vi "Handle Value Change.vi"(5 "VolatusAPI":refnum<class "VolatusAPI.lvclass">, 7 "CtlRef":refnum<vi>, 8 "error in (no error)":errorcluster, 9 "NewVal":variant, 10 "OldVal":variant, 11 "DigitalButtonControl in":refnum<class "DigitalButtonControl.lvclass">) -> (0 "error out":errorcluster, 3 "DigitalButtonControl out":refnum<class "DigitalButtonControl.lvclass">)   [LabVIEW 2023, in "VolatusGUIElements.lvlib" / "DigitalButtonControl.lvclass"]
uses:
  DigitalButtonControl.lvclass
  Volatus/VolatusAPI/VolatusAPI.lvclass
  messages/CmdDigital/Data.ctl
  DigitalButtonControl.lvclass/DigitalButtonControl.ctl
  messages/CmdDigital/Class/Msg.lvclass/Msg.ctl
  Volatus/VolatusAPI/VolatusAPI.lvclass/VolatusAPI.ctl
  messages/CmdDigital/Class/Msg.lvclass
  lv-vecto/Vecto/TCPMessageService/Send Message.vi
  <vilib>/Utility/error.llb/Error Cluster From Error Code.vi
  lv-protoc/LV-Proto/Message/Message.lvclass
  messages/CmdDigital/CmdDigital.lvlib
  VolatusGUI/GUI Element/GUI Element.lvclass
  messages/CmdDigitalMultiple/Class/Msg.lvclass
  C:/dev/volatus/mts-volatus-super/libs/lv-volatus/messages/CmdDigitalMultiple/Class/Msg.lvclass
  C:/dev/volatus/mts-volatus-super/libs/lv-protoc/LV-Proto/Message/Message.lvclass
  C:/dev/volatus/mts-volatus-super/libs/lv-volatus/VolatusGUI/GUI Element/GUI Element.lvclass
  C:/dev/volatus/mts-volatus-super/libs/lv-volatus/VolatusGUIElements/DigitalButtonControl/DigitalButtonControl.lvclass
  C:/dev/volatus/mts-volatus-super/libs/lv-volatus/VolatusGUI/OnValueChangeHandler/OnValueChangeHandler.lvclass
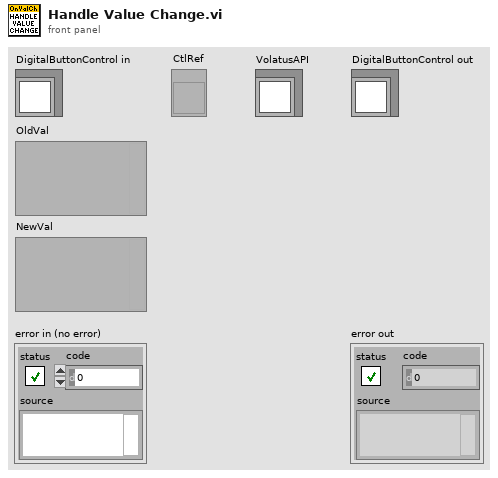
[diagram p1: front panel]
types:
  T1 = typedef "CmdDigital.lvlib/Data.ctl" = cluster{"channel":string, "value":bool}
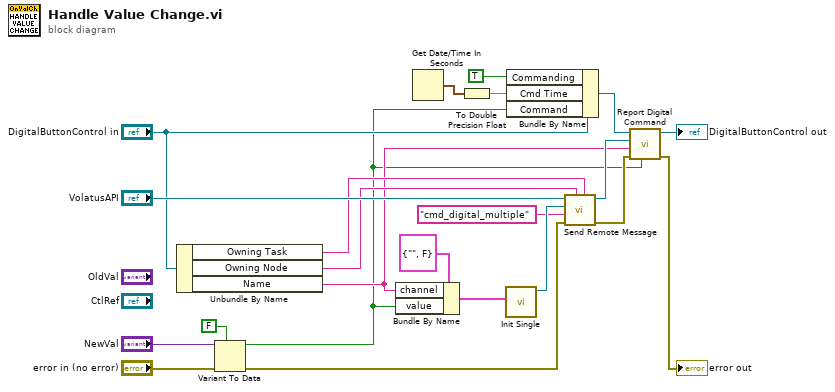
[diagram p0: block diagram]
diagram:
  n1 = Unbundle By Name("DigitalButtonControl in") -> ("Owning Task"=w8:string, "Owning Node"=w7:string, "Name"=w2:string)
  n2 = Variant To Data(error in="error in (no error)", type=FALSE, Variant="NewVal") -> (data=w1:bool, error out=w9:errorcluster)
  n3 = Bundle By Name(cluster=T1 {"channel"="", "value"=FALSE} ("Data"), "channel"=w2, "value"=w1) -> (w18:T1)
  n4 = Get Date/Time In Seconds() -> (seconds since 1Jan1904=w13:timestamp)
  n5 = To Double Precision Float(number=w13) -> (double precision float=w12:dbl)
  n6 = call "Init Single.vi"("value"=w18) -> ("Msg out"=w16:refnum<class "Msg.lvclass">)  [unwired: 10 in]
  n7 = Bundle By Name(cluster="DigitalButtonControl in", "Commanding"=TRUE, "Cmd Time"=w12, "Command"=w1) -> (w14:refnum<class "DigitalButtonControl.lvclass">)
  n8 = call "Send Remote Message.vi"("Target Task (None)"=w8, "Target Name"=w7, "error in (no error)"=w9, "Message Type"="cmd_digital_multiple", "Message"=w16, "VolatusAPI in"="VolatusAPI") -> ("error out"=w5:errorcluster, "VolatusAPI out"=w3:refnum<class "VolatusAPI.lvclass">)  [unwired: 4 in]
  n9 = call "Report Digital Command.vi"("Value"=w1, "error in (no error)"=w5, "Name"=w2, "VolatusAPI in"=w3, "GUI Element in"=w14) -> ("error out"=→"error out":errorcluster, "GUI Element out"=→"DigitalButtonControl out":refnum<class "DigitalButtonControl.lvclass">)  [unwired: 5 in]
